vi "Producer:Consumer.vi"() -> ()   [LabVIEW 2023]
panel:
  out "Histogram 2":dynamicdata(graph) caption="Histogram"
  in  "Stop Button 2":bool
  out "Waveform Chart 2":dbl(graph)
  out "Histogram":dynamicdata(graph)
  in  "Stop Button":bool
  out "Waveform Chart":dbl(graph)
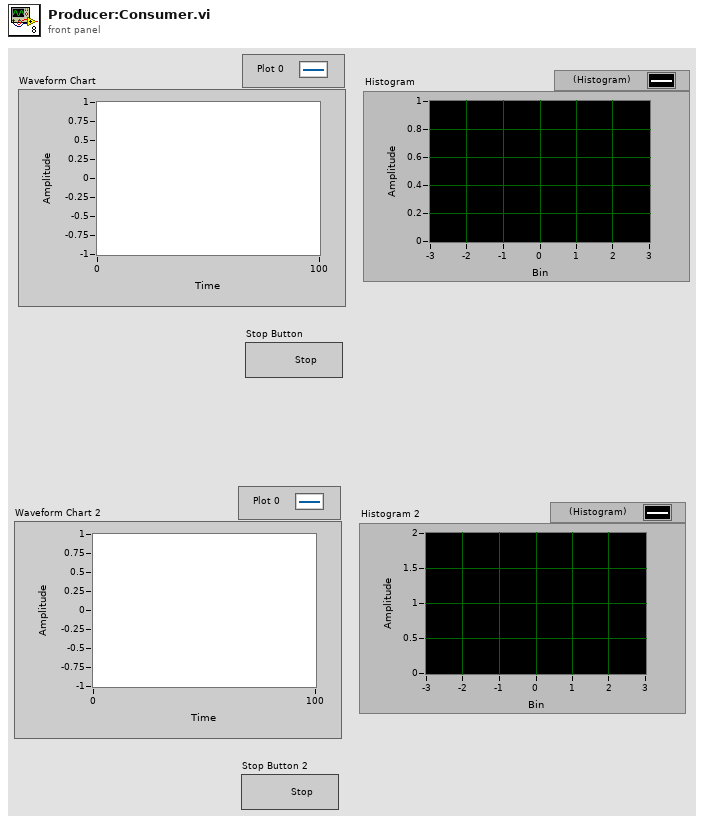
[diagram p1: front panel]
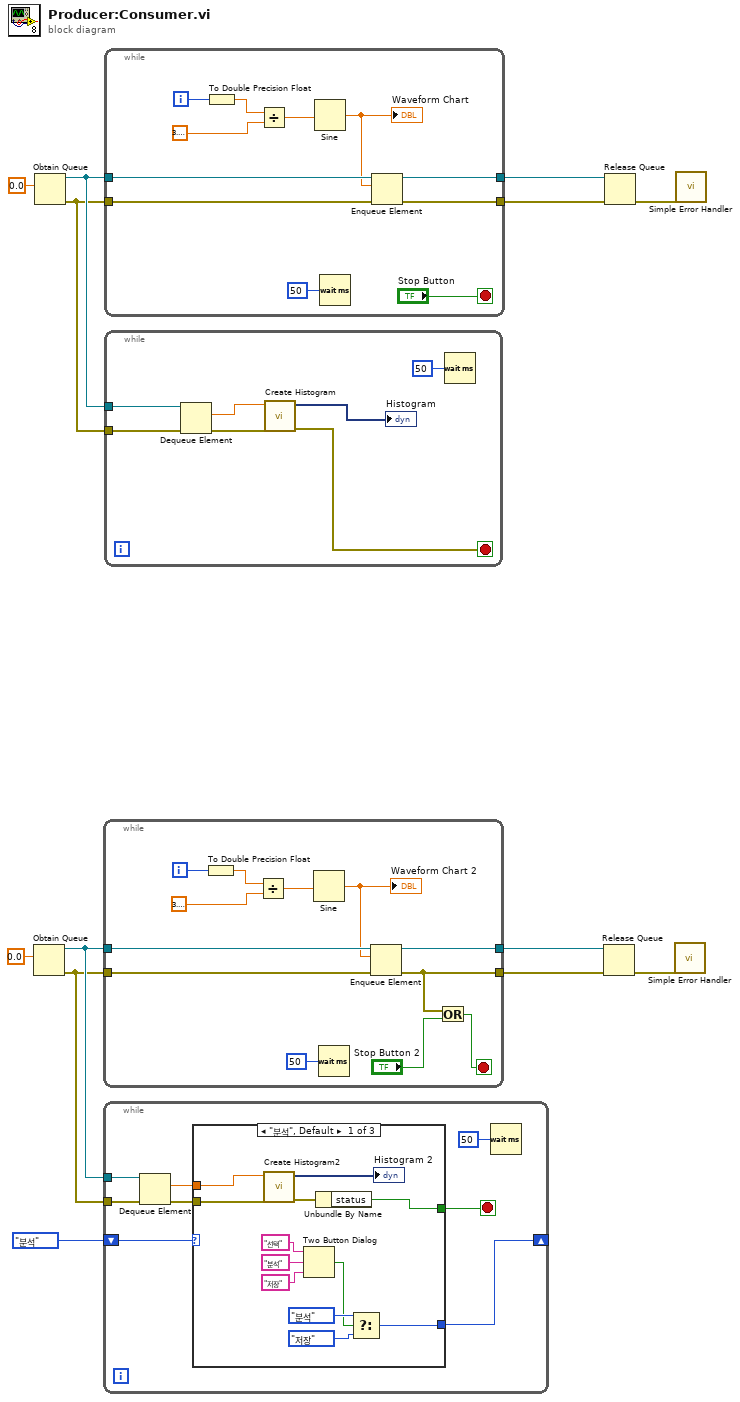
[diagram p0: block diagram]
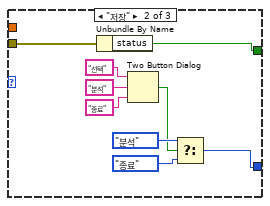
[diagram p2: hidden frame]
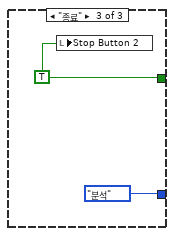
[diagram p3: hidden frame]
diagram:
  n1 = Obtain Queue(element data type=0.0) -> (queue out=w3:refnum<queue>, error out=w2:errorcluster)  [unwired: 4 in, 1 out]
  n2 = Obtain Queue(element data type=0.0) -> (queue out=w9:refnum<queue>, error out=w8:errorcluster)  [unwired: 4 in, 1 out]
  n3 = while {
    tunnel: [w16] -> w5
    tunnel: w2 -> [w20]
    tunnel: w3 -> [w19]
    tunnel: [w18] -> w4
    i -> [w25]
    stop <- w14 stop-if-true
    n4 = To Double Precision Float(number=w25) -> (double precision float=w24:dbl)
    n5 = Divide(x=w24, y=3.141592653589793) -> (x/y=w21:dbl)
    n6 = Sine(x=w21) -> (sin(x)=w17:dbl)
    "Waveform Chart 2" <- w17
    n7 = Wait (ms)(milliseconds to wait=u32 50) -> ()  [unwired: 1 out]
    n8 = Enqueue Element(queue=w19, element=w17, error in (no error)=w20) -> (queue out=w18:refnum<queue>, error out=w16:errorcluster)  [unwired: 1 in, 1 out]
    n9 = Or(x=w16, y="Stop Button 2") -> (x .or. y?=w14:bool)
  }
  n10 = while {
    tunnel: w3 -> [w33]
    tunnel: w2 -> [w32]
    shift-right: [w26] -> _
    shift-left: enum16{"분석", "저장", "종료"}."분석" -> [w27]
    stop <- w30 stop-if-true
    n11 = Dequeue Element(queue=w33, error in (no error)=w32) -> (element=w28:dbl, error out=w31:errorcluster)  [unwired: 1 in, 2 out]
    n12 = case shown="\"분석\", Default" w27 {
      tunnel: w31 -> [w45 w54 _]
      tunnel: [w41 w53 w55] -> w30
      tunnel: w28 -> [w43 _ _]
      tunnel: [w34 w46 enum16{"분석", "저장", "종료"}."분석"] -> w26
      frame "분석", Default {
        n13 = call "Create Histogram2"("error in (no error)"=w45, "Signal"=w43) -> ("error out"=w42:errorcluster, "Histogram"=→"Histogram 2":dynamicdata)  [unwired: 8 in]
        n14 = Two Button Dialog(message="선택", 1:"저장" ("F button name (\"Cancel\")"), 2:"분석" ("T button name (\"OK\")")) -> (T button?=w35:bool)
        n15 = Unbundle By Name(w42) -> ("status"=w41:bool)
        n16 = Select(t=enum16{"분석", "저장", "종료"}."분석", s=w35, f=enum16{"분석", "저장", "종료"}."저장") -> (s? t:f=w34:enum16{"분석", "저장", "종료"})
      }
      frame "저장" {
        n17 = Unbundle By Name(w54) -> ("status"=w53:bool)
        n18 = Two Button Dialog(message="선택", 1:"종료" ("F button name (\"Cancel\")"), 2:"분석" ("T button name (\"OK\")")) -> (T button?=w47:bool)
        n19 = Select(t=enum16{"분석", "저장", "종료"}."분석", s=w47, f=enum16{"분석", "저장", "종료"}."종료") -> (s? t:f=w46:enum16{"분석", "저장", "종료"})
      }
      frame "종료" {
        w55 = TRUE
        n20 = local write "Stop Button 2"(w55) -> ()
      }
    }
    n21 = Wait (ms)(milliseconds to wait=u32 50) -> ()  [unwired: 1 out]
  }
  n22 = while {
    tunnel: [w61] -> w11
    tunnel: w8 -> [w60]
    tunnel: w9 -> [w59]
    tunnel: [w58] -> w10
    i -> [w67]
    stop <- "Stop Button" stop-if-true
    n23 = To Double Precision Float(number=w67) -> (double precision float=w66:dbl)
    n24 = Divide(x=w66, y=3.141592653589793) -> (x/y=w62:dbl)
    n25 = Sine(x=w62) -> (sin(x)=w57:dbl)
    "Waveform Chart" <- w57
    n26 = Wait (ms)(milliseconds to wait=u32 50) -> ()  [unwired: 1 out]
    n27 = Enqueue Element(queue=w59, element=w57, error in (no error)=w60) -> (queue out=w58:refnum<queue>, error out=w61:errorcluster)  [unwired: 1 in, 1 out]
  }
  n28 = while {
    tunnel: w9 -> [w74]
    tunnel: w8 -> [w73]
    stop <- w71 stop-if-true
    n29 = Dequeue Element(queue=w74, error in (no error)=w73) -> (element=w68:dbl, error out=w72:errorcluster)  [unwired: 1 in, 2 out]
    n30 = call "Create Histogram"("error in (no error)"=w72, "Signal"=w68) -> ("error out"=w71:errorcluster, "Histogram"=→"Histogram":dynamicdata)  [unwired: 8 in]
    n31 = Wait (ms)(milliseconds to wait=u32 50) -> ()  [unwired: 1 out]
  }
  n32 = Release Queue(queue=w4, error in (no error)=w5) -> (error out=w6:errorcluster)  [unwired: 1 in, 2 out]
  n33 = Release Queue(queue=w10, error in (no error)=w11) -> (error out=w12:errorcluster)  [unwired: 1 in, 2 out]
  n34 = call <vilib>:"Simple Error Handler.vi"("error in (no error)"=w6) -> ()  [unwired: 4 in, 5 out]
  n35 = call <vilib>:"Simple Error Handler.vi"("error in (no error)"=w12) -> ()  [unwired: 4 in, 5 out]
